vi "merge_two_y_axes.vi"(8 "X":dbl[](array[numeric]), 10 "Y2":dbl[](array[numeric]), 11 "Y1":dbl[](array[numeric])) -> (0 "graph_data":cluster{"Y":dbl[], "X2":dbl[]}[](array[cluster]))   [LabVIEW 2025]
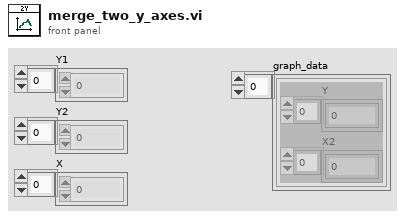
[diagram p1: front panel]
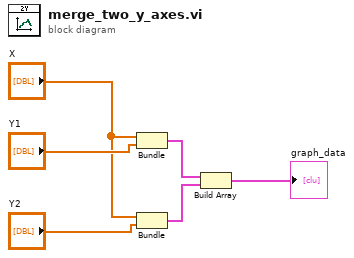
[diagram p0: block diagram]
diagram:
  n1 = Bundle("X"="X", "Y1"="Y1") -> (w6:cluster{"X":dbl[], "Y1":dbl[]})  [unwired: 1 in]
  n2 = Bundle("X"="X", "Y2"="Y2") -> (w5:cluster{"X":dbl[], "Y2":dbl[]})  [unwired: 1 in]
  n3 = Build Array(w6, w5) -> (→"graph_data":cluster{"X":dbl[], "Y2":dbl[]}[])
